vi "Get Buffer Statistics.vi"(0 "VISA resource name":refnum<visa-resource-name>, 5 "Buffer Name (defbuffer1)":string="defbuffer1", 7 "Statistics Type":i32(ring) items=["Average", "Maximum", "Minimum", "Peak-to-peak", "Standard deviation"], 11 "error in (no error)":errorcluster) -> (4 "VISA resource name out":refnum<visa-resource-name>, 8 "Statistics Value":dbl, 15 "error out":errorcluster)   [LabVIEW 2016, in "Keithley DMM7510.lvlib"]
doc: "This clears the statistical information associated with the specified buffer."
uses:
  Keithley DMM7510.lvlib
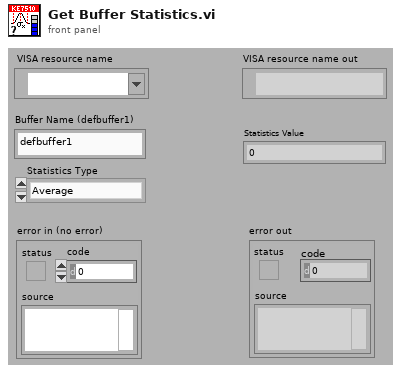
[diagram p1: front panel]
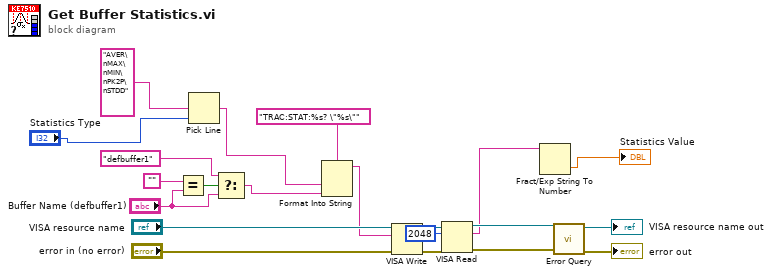
[diagram p0: block diagram]
diagram:
  n1 = Equal?(x="", y="Buffer Name (defbuffer1)") -> (x = y?=w19:bool)
  n2 = Pick Line(multi-line string="AVER\nMAX\nMIN\nPK2P\nSTDD", line index="Statistics Type") -> (output string=w2:string)  [unwired: 1 in]
  n3 = Select(t="defbuffer1", s=w19, f="Buffer Name (defbuffer1)") -> (s? t:f=w1:string)
  n4 = Format Into String(format string="TRAC:STAT:%s? \"%s\"" ("Read Measurement"), w2, w1) -> (resulting string=w12:string)  [unwired: 2 in, 1 out]
  n5 = VISA Write(VISA resource name="VISA resource name", write buffer=w12, error in (no error)="error in (no error)") -> (VISA resource name out=w9:refnum<visa-resource-name>, error out=w8:errorcluster)  [unwired: 1 out]
  n6 = VISA Read(VISA resource name=w9, byte count=u32 2048, error in (no error)=w8) -> (VISA resource name out=w7:refnum<visa-resource-name>, read buffer=w4:string, error out=w6:errorcluster)  [unwired: 1 out]
  n7 = Fract/Exp String To Number(string=w4) -> (number=→"Statistics Value":dbl)  [unwired: 3 in, 1 out]
  n8 = call "Error Query.vi"("error in (no error)"=w6, "VISA resource name"=w7) -> ("error out"=→"error out":errorcluster, "VISA resource name out"=→"VISA resource name out":refnum<visa-resource-name>)  [unwired: 8 out]
